vi "validate key value pair.vi"(8 "error in":errorcluster, 9 "value":string, 10 "key":string, 11 "GPIC ScaleAndLimit configuration in":refnum<class "GPIC ScaleAndLimit configuration.lvclass">) -> (0 "error out":errorcluster, 3 "GPIC ScaleAndLimit configuration out":refnum<class "GPIC ScaleAndLimit configuration.lvclass">)   [LabVIEW 2015, in "GPIC ScaleAndLimit configuration.lvclass"]
uses:
  GPIC ScaleAndLimit configuration.lvclass
  <vilib>/NI/DCAF/Tag Editor Core/control module/configuration/control module configuration.lvclass
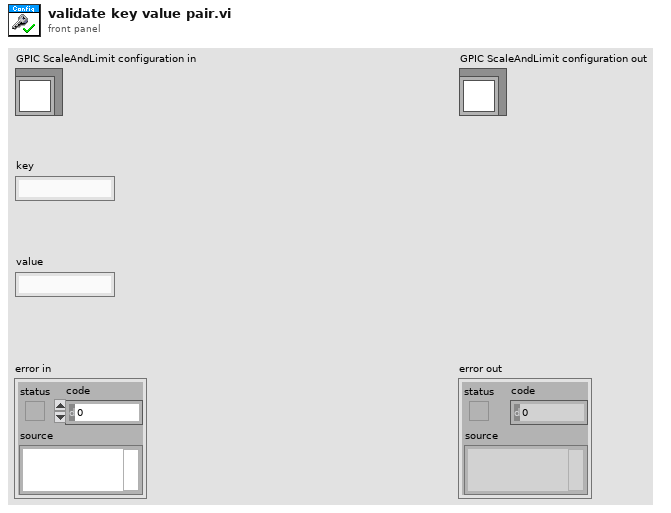
[diagram p1: front panel]
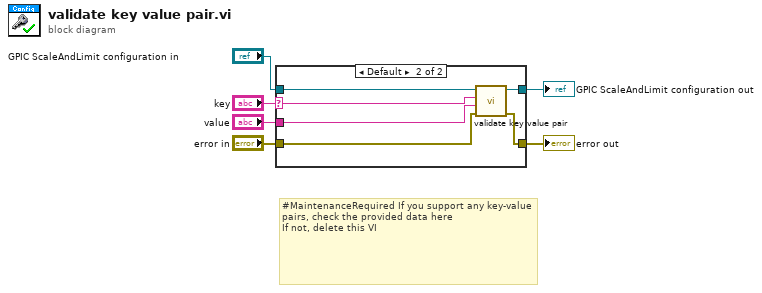
[diagram p0: block diagram]
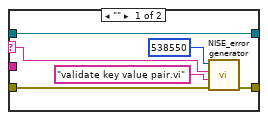
[diagram p2: hidden frame]
diagram:
  # "#MaintenanceRequired If you support any key-value pairs, check the provided data here\nIf not, delete this VI"
  n1 = case shown="Default" "key" {
    selector: "key" -> [w9 w13]
    tunnel: [w7 w18] -> w6
    tunnel: [w12 w17] -> w5
    tunnel: "error in" -> [w8 w16]
    tunnel: "value" -> [_ w15]
    tunnel: "GPIC ScaleAndLimit configuration in" -> [w12 w14]
    frame "" {
      n2 = call <vilib>:"NISE_error generator.vi"("error in"=w8, "source"="validate key value pair.vi", "append error message"=w9, "error code (0)"=538550) -> ("error out"=w7:errorcluster)  [unwired: 5 in]
    }
    frame Default {
      n3 = call-parent "validate key value pair.vi"("error in"=w16, "value"=w15, "key"=w13, "fixed channel configuration in"=w14) -> ("error out"=w18:errorcluster, "fixed channel configuration out"=w17:refnum<class "GPIC ScaleAndLimit configuration.lvclass">)  [unwired: 6 in]
    }
  }
  "error out" <- w6
  "GPIC ScaleAndLimit configuration out" <- w5
